vi "test7-AsyncMessageWithoutReply.vi"(8 "error in (no error)":errorcluster, 11 "TestCase in":refnum<class "testcase-CSMMessage.lvclass">) -> (0 "error out":errorcluster, 3 "TestCase out":refnum<class "testcase-CSMMessage.lvclass">)   [LabVIEW 2017, in "testcase-CSMMessage.lvclass"]
uses:
  testcase-CSMMessage.lvclass
  7412589e-de49-4983-aece-358686b48526.vi
  <vilib>/addons/_JKI Toolkits/VI Tester/TestCase.llb/TestCase.lvclass
  src/user.lib/_NEVSTOP/Communicable State Machine(CSM)/Communicable State Machine.lvlib
  C:/Program Files (x86)/National Instruments/LabVIEW 2017/vi.lib/addons/_JKI Toolkits/VI Tester/TestCase.llb/TestCase.lvclass
panel:
  out "Loop count":i32
  out "debug message":string
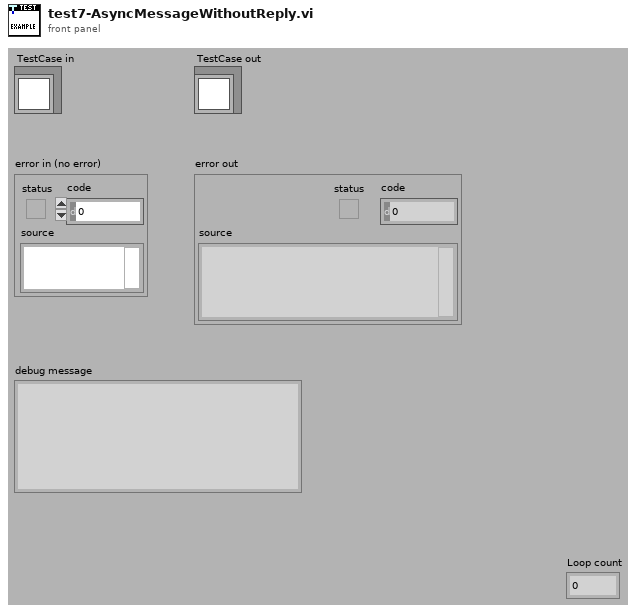
[diagram p1: front panel]
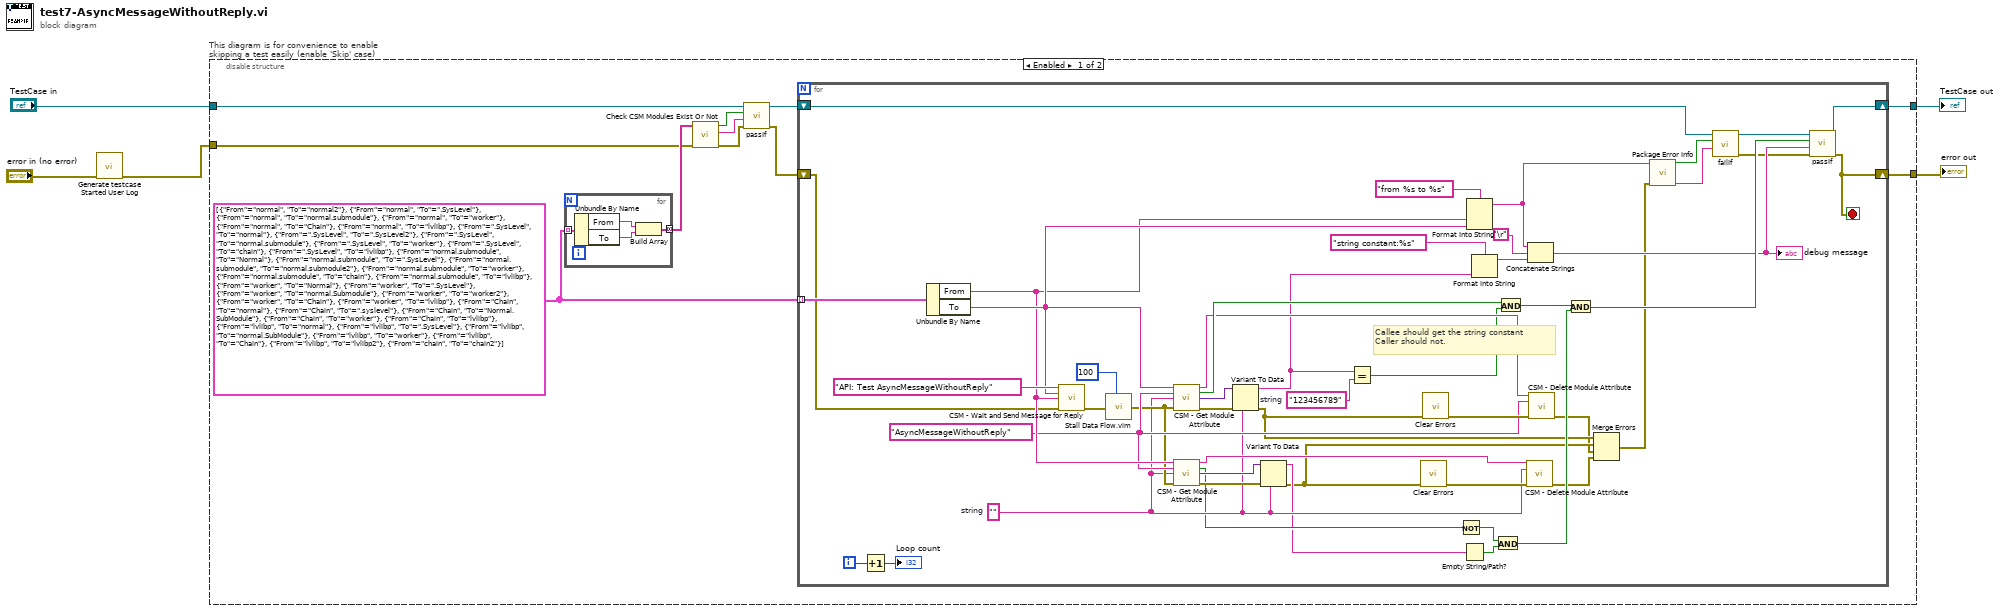
[diagram p0: block diagram]
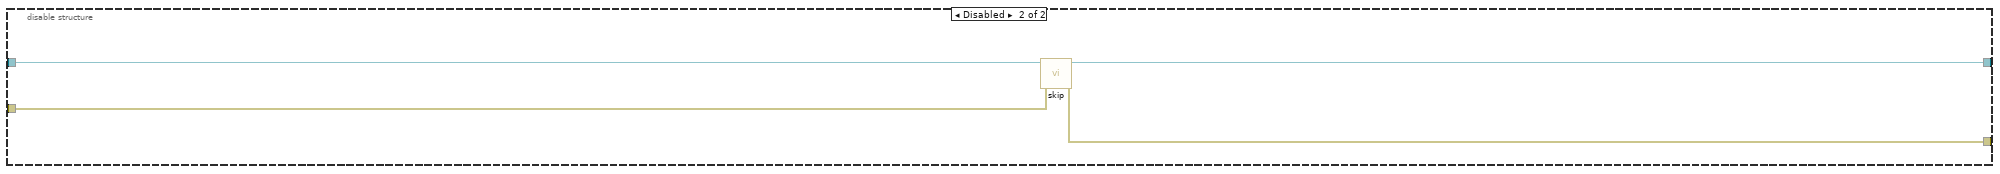
[diagram p2: hidden frame]
diagram:
  n1 = call "Generate testcase Started User Log.vi"("Error In"="error in (no error)") -> ("error out"=w1:errorcluster)  [unwired: 10 in]
  n2 = disable-structure "This diagram is for convenience to enable skipping a test easily (enable 'Skip' case)" shown="Enabled" {
    disable-tunnel: "TestCase in" -> [w9 w73]
    disable-tunnel: [w7 w71] -> w2
    disable-tunnel: [w6 w72] -> w4
    disable-tunnel: w1 -> [w11 w70]
    frame Enabled {
      w12 = cluster{"From":string, "To":string}[] [{"From"="normal", "To"="normal2"}, {"From"="normal", "To"=".SysLevel"}, {"From"="normal", "To"="normal.submodule"}, {"From"="normal", "To"="worker"}, {"From"="normal", "To"="Chain"}, {"From"="normal", "To"="lvlibp"}, {"From"=".SysLevel", "To"="normal"}, {"From"=".SysLevel", "To"=".SysLevel2"}, {"From"=".SysLevel", "To"="normal.submodule"}, {"From"=".SysLevel", "To"="worker"}, {"From"=".SysLevel", "To"="chain"}, {"From"=".SysLevel", "To"="lvlibp"}, {"From"="normal.submodule", "To"="Normal"}, {"From"="normal.submodule", "To"=".SysLevel"}, {"From"="normal.submodule", "To"="normal.submodule2"}, {"From"="normal.submodule", "To"="worker"}, {"From"="normal.submodule", "To"="chain"}, {"From"="normal.submodule", "To"="lvlibp"}, {"From"="worker", "To"="Normal"}, {"From"="worker", "To"=".SysLevel"}, {"From"="worker", "To"="normal.Submodule"}, {"From"="worker", "To"="worker2"}, {"From"="worker", "To"="Chain"}, {"From"="worker", "To"="lvlibp"}, {"From"="Chain", "To"="normal"}, {"From"="Chain", "To"=".syslevel"}, {"From"="Chain", "To"="Normal.SubModule"}, {"From"="Chain", "To"="worker"}, {"From"="Chain", "To"="lvlibp"}, {"From"="lvlibp", "To"="normal"}, {"From"="lvlibp", "To"=".SysLevel"}, {"From"="lvlibp", "To"="normal.SubModule"}, {"From"="lvlibp", "To"="worker"}, {"From"="lvlibp", "To"="Chain"}, {"From"="lvlibp", "To"="lvlibp2"}, {"From"="chain", "To"="chain2"}]
      n3 = for {
        tunnel: w12 -> [w20] mode=indexing
        tunnel: [w17] -> w15 mode=concatenating
        n4 = Unbundle By Name(w20) -> ("From"=w19:string, "To"=w18:string)
        n5 = Build Array(w19, w18) -> (w17:string[])
      }
      n6 = call "Check CSM Modules Exist Or Not.vi"("error in"=w11, "CSM names in"=w15) -> ("error out"=w13:errorcluster, "Debug string"=w14:string, "All Modules Exist?"=w16:bool)  [unwired: 7 in]
      n7 = call-dynamic "passIf.vi"("error in (no error)"=w13, "message (\"\")"=w14, "pass"=w16, "TestCase in"=w9) -> ("error out"=w10:errorcluster, "TestCase out"=w8:refnum<class "testcase-CSMMessage.lvclass">)  [unwired: 6 in]
      n8 = for {
        tunnel: w12 -> [w64] mode=indexing
        shift-right: [w69] -> w7
        shift-left: w8 -> [w25]
        shift-right: [w57] -> w6
        shift-left: w10 -> [w33]
        i -> [w37]
        stop <- w57 stop-if-true
        w54 = "123456789"  # string
        w45 = ""  # string
        w51 = "AsyncMessageWithoutReply" ("State With Arguments")
        # "Callee should get the string constant\nCaller should not."
        n9 = Increment(x=w37) -> (x+1=→"Loop count":i32)
        n10 = Unbundle By Name(w64) -> ("From"=w52:string, "To"=w56:string)
        n11 = call "CSM - Wait and Send Message for Reply.vi"("State"="API: Test AsyncMessageWithoutReply", "Arguments (\"\")"=w56, "Target Module"=w52, "Error In (No Error)"=w33) -> ("error out"=w35:errorcluster)  [unwired: 8 in, 3 out]
        n12 = call "Stall Data Flow.vim"("value in"=w35, "milliseconds to wait"=u32 100) -> ("value out"=w50:errorcluster)  [unwired: 1 out]
        n13 = call "CSM - Get Module Attribute.vi"("CSM Name"=w56, "Attribute"=w51, "Default Value (Empty Variant)"=w45, "Error In"=w50) -> ("CSM Name (Dup)"=w62:string, "Found"=w65:bool, "Value"=w66:variant, "error out"=w67:errorcluster)  [unwired: 7 in, 1 out]
        n14 = call "CSM - Get Module Attribute.vi"("CSM Name"=w52, "Attribute"=w51, "Default Value (Empty Variant)"=w45, "Error In"=w50) -> ("CSM Name (Dup)"=w46:string, "Found"=w44:bool, "Value"=w47:variant, "error out"=w49:errorcluster)  [unwired: 7 in, 1 out]
        n15 = Variant To Data(error in=w67, type=w45, Variant=w66) -> (data=w53:string, error out=w32:errorcluster)
        n16 = Variant To Data(error in=w49, type=w45, Variant=w47) -> (data=w43:string, error out=w31:errorcluster)
        n17 = Equal?(x=w53, y=w54) -> (x = y?=w55:bool)
        n18 = call <vilib>:"Clear Errors.vi"("error in (no error)"=w31) -> ("error out"=w48:errorcluster)  [unwired: 5 in, 1 out]
        n19 = call <vilib>:"Clear Errors.vi"("error in (no error)"=w32) -> ("error out"=w58:errorcluster)  [unwired: 5 in, 1 out]
        n20 = Not(x=w44) -> (.not. x?=w40:bool)
        n21 = Empty String/Path?(string/path=w43) -> (empty?=w42:bool)
        n22 = Format Into String(format string="from %s to %s", w52, w56) -> (resulting string=w21:string)  [unwired: 2 in, 1 out]
        n23 = Format Into String(format string="string constant:%s", w53) -> (resulting string=w61:string)  [unwired: 2 in, 1 out]
        n24 = And(x=w40, y=w42) -> (x .and. y?=w38:bool)
        n25 = And(x=w65, y=w55) -> (x .and. y?=w41:bool)
        n26 = call "CSM - Delete Module Attribute.vi"("CSM Name"=w46, "Attribute"=w45, "Error In"=w48) -> ("error out"=w29:errorcluster)  [unwired: 9 in, 3 out]
        n27 = Concatenate Strings(w21, "\r", w61) -> (w28:string)
        "debug message" <- w28
        n28 = call "CSM - Delete Module Attribute.vi"("CSM Name"=w62, "Attribute"=w51, "Error In"=w58) -> ("error out"=w30:errorcluster)  [unwired: 9 in, 3 out]
        n29 = And(x=w41, y=w38) -> (x .and. y?=w39:bool)
        n30 = Merge Errors(w32, w31, w30, w29) -> (w22:errorcluster)
        n31 = call "Package Error Info.vi"("error in"=w22, "String in"=w21) -> ("packed error info out"=w26:string, "error status"=w27:bool)  [unwired: 8 in]
        n32 = call-dynamic "failIf.vi"("message (\"\")"=w26, "fail"=w27, "TestCase in"=w25) -> ("error out"=w23:errorcluster, "TestCase out"=w24:refnum<class "testcase-CSMMessage.lvclass">)  [unwired: 7 in]
        n33 = call-dynamic "passIf.vi"("error in (no error)"=w23, "message (\"\")"=w28, "pass"=w39, "TestCase in"=w24) -> ("error out"=w57:errorcluster, "TestCase out"=w69:refnum<class "testcase-CSMMessage.lvclass">)  [unwired: 6 in]
      }
    }
    frame Disabled {
      # "skip test result while test is under development"
      n34 = call <vilib>:"skip.vi"("error in (no error)"=w70, "TestCase in"=w73) -> ("error out"=w72:errorcluster, "TestCase out"=w71:refnum<class "testcase-CSMMessage.lvclass">)  [unwired: 8 in]
    }
  }
  "error out" <- w4
  "TestCase out" <- w2
